vi "Read Set output.vi"(8 "error in (no error)":errorcluster, 11 "Set Sweep in":refnum<class "Set Sweep.lvclass">) -> (0 "error out":errorcluster, 2 "Set output":T1={"Set point"=0.0, "Sweep rate"=0.1, "Sweep action"=enum."To set point"}, 3 "Set Sweep out":refnum<class "Set Sweep.lvclass">)   [LabVIEW 2018, in "Set Sweep.lvclass"]
uses:
  Set Sweep.lvclass
  Controls/Set Output.ctl
  Controls/Sweep Action.ctl
  Set Sweep.lvclass/Set Sweep.ctl
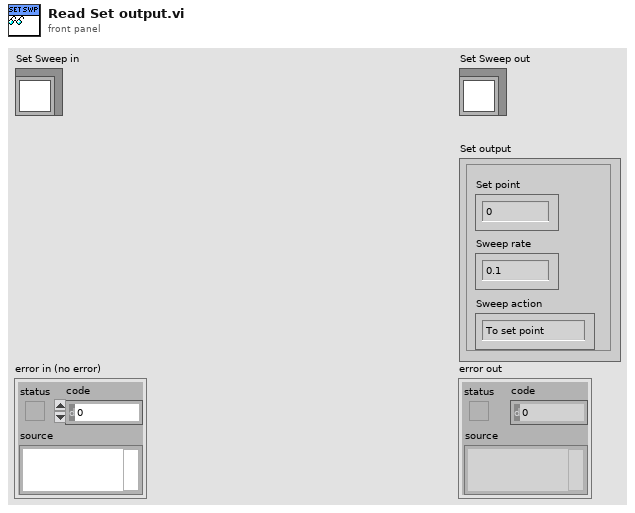
[diagram p1: front panel]
types:
  T1 = typedef "Set Output.ctl" = cluster{"Set point":dbl, "Sweep rate":dbl, "Sweep action":T2}
  T2 = typedef "Sweep Action.ctl" = enum16{"To set point", "To zero", "Hold", "Clamp"}
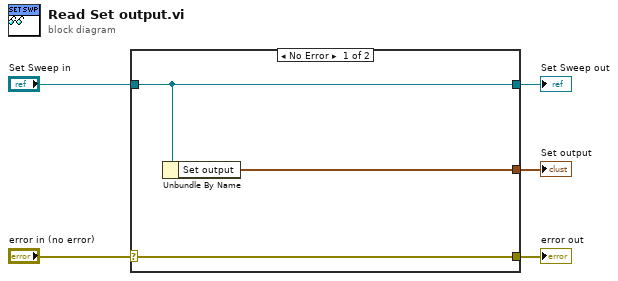
[diagram p0: block diagram]
diagram:
  n1 = case shown="No Error" "error in (no error)" {
    selector: "error in (no error)" -> [w8 w9]
    tunnel: [w8 w9] -> w4
    tunnel: [w7 w10] -> w2
    tunnel: "Set Sweep in" -> [w7 w10]
    tunnel: [w6 _] -> w1
    frame No Error {
      n2 = Unbundle By Name(w7) -> ("Set output"=w6:T1)
    }
    frame Error {
    }
  }
  "error out" <- w4
  "Set Sweep out" <- w2
  "Set output" <- w1
